vi "make_node.vi"(0 "VIName":string, 1 "VIPath":string, 2 "id":string, 3 "type":string, 4 "label":string, 5 "parentId":string, 6 "properties":variant[](array[variant]), 7 "metadata":variant[](array[variant]), 8 "frames":variant[](array[variant]), 9 "nodes":variant[](array[variant]), 10 "terminals":T1[](array[typedef]), 11 "name":string) -> (14 "node":T4)   [LabVIEW 2020]
uses:
  node.ctl
  terminalData.ctl
  terminal_type.ctl
  terminal_direction.ctl
panel:
  # "tunnel/judge/shift?"
  # "tunnel/judge/shift?"
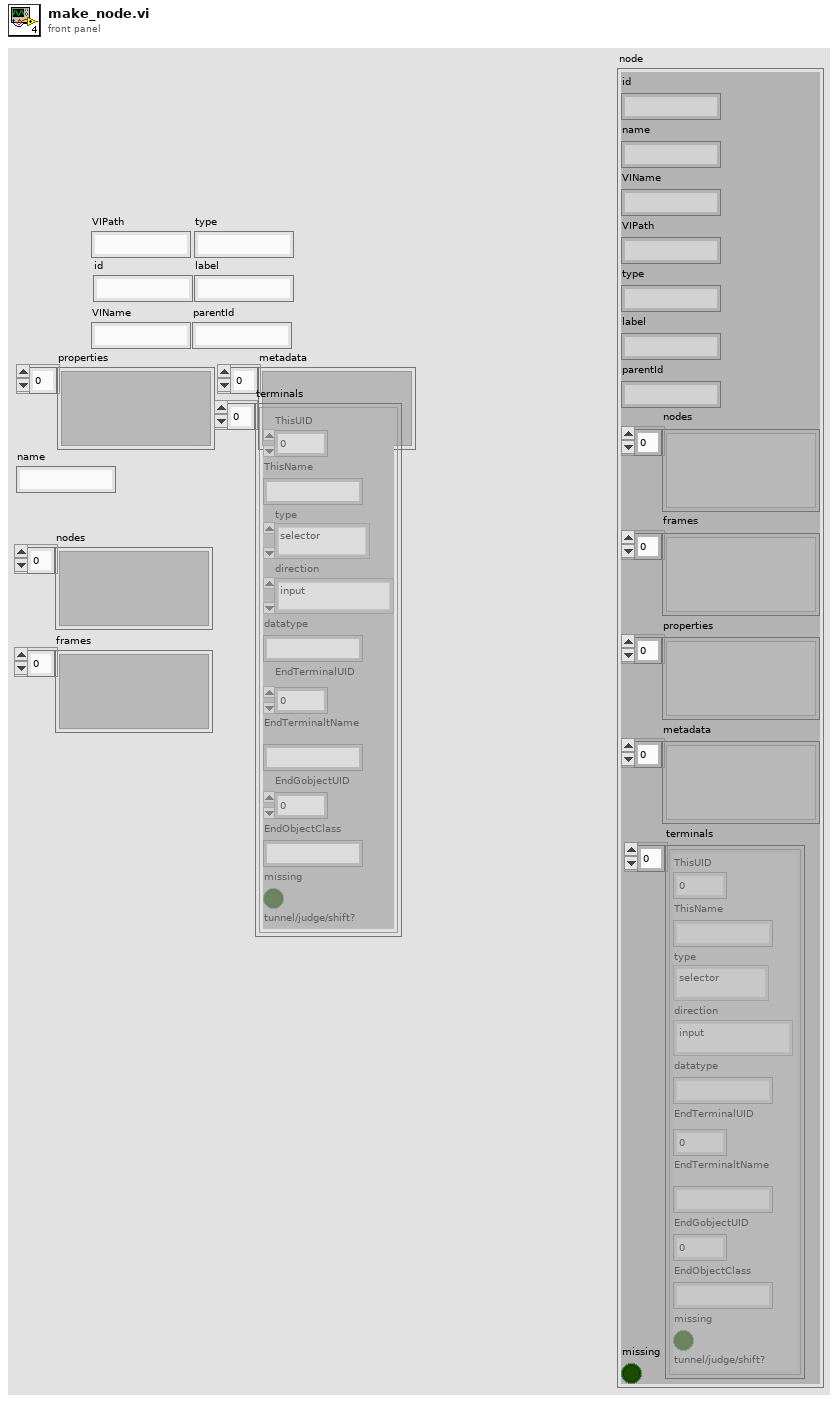
[diagram p1: front panel]
types:
  T1 = typedef "terminalData.ctl" = cluster{"ThisUID":i32, "ThisName":string, "type":T2, "direction":T3, "datatype":string, "EndTerminalUID":i32, "EndTerminaltName":string, "EndGobjectUID":i32, "EndObjectClass":string, "missing":bool}
  T2 = typedef "terminal_type.ctl" = enum16{"selector", "tunnel", "shift", "timeout", "normal", "floating"}
  T3 = typedef "terminal_direction.ctl" = enum16{"input", "output"}
  T4 = typedef "node.ctl" = cluster{"id":string, "name":string, "VIName":string, "VIPath":string, "type":string, "label":string, "parentId":string, "nodes":variant[], "frames":variant[], "properties":variant[], "metadata":variant[], "terminals":T1[], "missing":bool}
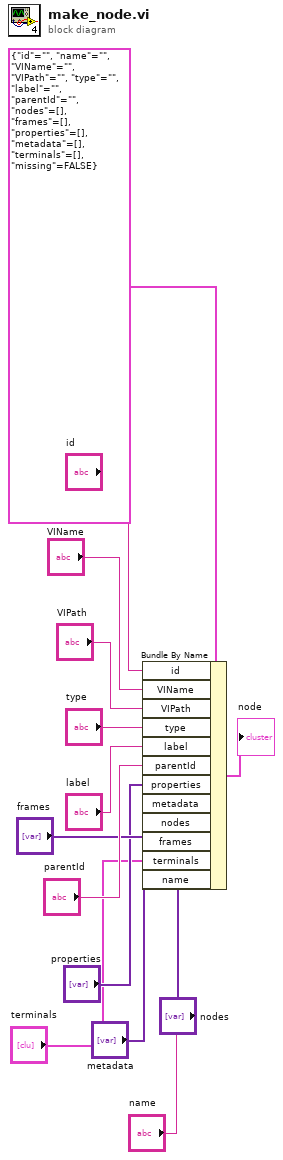
[diagram p0: block diagram]
diagram:
  n1 = Bundle By Name(cluster=T4 {"id"="", "name"="", "VIName"="", "VIPath"="", "type"="", "label"="", "parentId"="", "nodes"=[], "frames"=[], "properties"=[], "metadata"=[], "terminals"=[], "missing"=FALSE} ("node_cluster"), "id"="id", "VIName"="VIName", "VIPath"="VIPath", "type"="type", "label"="label", "parentId"="parentId", "properties"="properties", "metadata"="metadata", "nodes"="nodes", "frames"="frames", "terminals"="terminals", "name"="name") -> (→"node":T4)
